vi "RTTrapTest-05-2017.vi"() -> ()   [LabVIEW 2010]
uses:
  <vilib>/rvi/interface/nirviOpenFPGA/nirviOpenFPGA.xnode
  <vilib>/userDefined/High Color/nirio_resource_hc.ctl
  <vilib>/rvi/interface/nirviReadWriteControl/nirviReadWriteControl.xnode
  <vilib>/Utility/error.llb/Error Cluster From Error Code.vi
  <vilib>/rvi/errors/niLvFpgaWhatHappensToTopLevelVI.ctl
  <vilib>/rvi/interface/common/niFpgaNodeNameForErrorReporting.ctl
  <vilib>/rvi/errors/niLvFpgaAdjustHostInterfaceError.vi
  <vilib>/rvi/interface/nirviMethod/nirviMethod.xnode
  NiFpgaLv.dll
  <vilib>/rvi/interface/nirviCloseFPGA/nirviCloseFPGA.xnode
  C:/Users/HAGAR-IV/Desktop/Zeugs/markus/version feb 2012/FPGA Bitfiles/pertrasgcfpga2_FPGATarget_FPGA-TrapTest-05_C2F74D86.lvbitx
  C:/Users/HAGAR-IV/Desktop/Zeugs/Johnny/pertrasgc fpga/FPGA-TrapTest-05-2017.vi
  <vilib>/FPGAPlugInAG/cRIO-9114/niLvFpga_Open_cRIO-9114.vi
  <vilib>/rvi/ClientSDK/nirviWhatTheDeviceIsDoing.ctl
  <vilib>/RVI Host/nirviSupport.llb/nirviErrorClusterFromErrorCode.vi
  <vilib>/FPGAPlugInAG/cRIO-9114/niLvFpga_Close_cRIO-9114.vi
panel:
  in  "Vorlaufzeit":dbl
  in  "Heizung aus":bool
  out "Uhr":dbl
  in  "Heizen&Starten":bool
  in  "Rampenende":dbl
  in  "T2":dbl
  in  "T1":dbl
  out "ThermoTemp":dbl
  out "PTTempTrap":dbl[](graph)
  in  "ThermoKoeff0":dbl=12.98
  in  "ThermoKoeff2":dbl=-136.78
  in  "ThermoKoeff1":dbl=1284.53
  in  "PTStirlingKoeff0":dbl=-248.3
  in  "PTStirlingKoeff2":dbl=2.42
  in  "PTStirlingKoeff1":dbl=108.05
  in  "SollwertTemp":dbl=50.0
  in  "R(T)Koeff0":dbl=7.31
  in  "R(T)Koeff2":dbl=5.2e-05
  in  "R(T)Koeff1":dbl=0.032
  out "TempTrap":dbl[](graph)
  in  "Löschen":bool
  out "SollwertSchpannung":dbl
  out "SollwertWidrschtond":dbl=8.43
  out "TempTrap":dbl
  in  "T(R)Koeff0":dbl=-236.6
  in  "T(R)Koeff2":dbl=-0.6
  in  "T(R)Koeff1":dbl=37.1
  out "WiderstandHeizdraht":dbl
  out "PTStirling":dbl format="%.2f"
  in  "Stirling":bool
  out "Thermo [V]":fxp<+/-,26,5> format="%.23g"
  in  "Messwerte":i32=10
  in  "Heizen":bool
  in  "5Van(us)":u16=5500
  in  "Periode(us)":u32=100000
  out "Messwert":fxp<+/-,27,6> format="%.23g"
  in  "Warten(us)":u16=5000
  in  "zwischenMesswerten(us)":u16=10
  in  "PID gains":T1={"proportional gain (Kc)"=5.0, "integral gain (Kc*Ts/Ti)"=0.0, "derivative gain (Kc*Td/Ts)"=0.0} {"proportional gain (Kc)" format="%.11g"; "integral gain (Kc*Ts/Ti)" format="%.11g"; "derivative gain (Kc*Td/Ts)" format="%.11g"}
  in  "stop":bool
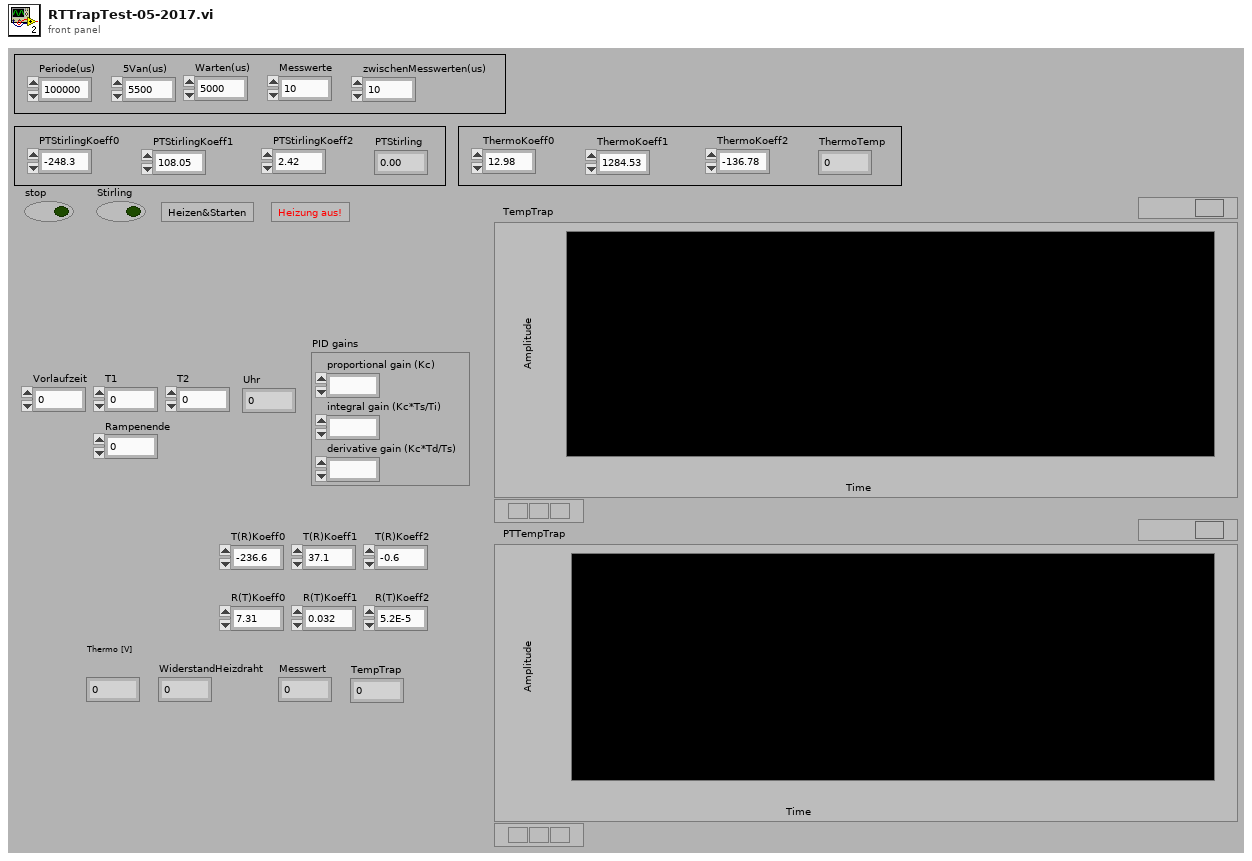
[diagram p1: front panel]
types:
  T1 = cluster{"proportional gain (Kc)":fxp<+/-,16,8>, "integral gain (Kc*Ts/Ti)":fxp<+/-,16,8>, "derivative gain (Kc*Td/Ts)":fxp<+/-,16,8>}
  T2 = typedef "niFpgaNodeNameForErrorReporting.ctl" = enum16{"Open FPGA VI Reference", "Read/Write Control", "Invoke Method: Abort", "Invoke Method: Acknowledge IRQ", "Invoke Method: Download", "Invoke Method: FIFO.Configure", "Invoke Method: FIFO.Read", "Invoke Method: FIFO.Start", "Invoke Method: FIFO.Stop", "Invoke Method: FIFO.Write", "Invoke Method: Reset", "Invoke Method: Run", "Invoke Method: Wait on IRQ", "Close FPGA VI Reference"}
  T3 = typedef "niLvFpgaWhatHappensToTopLevelVI.ctl" = enum16{"top level VI scripted behind XNode", "top level VI inlined behind XNode"}
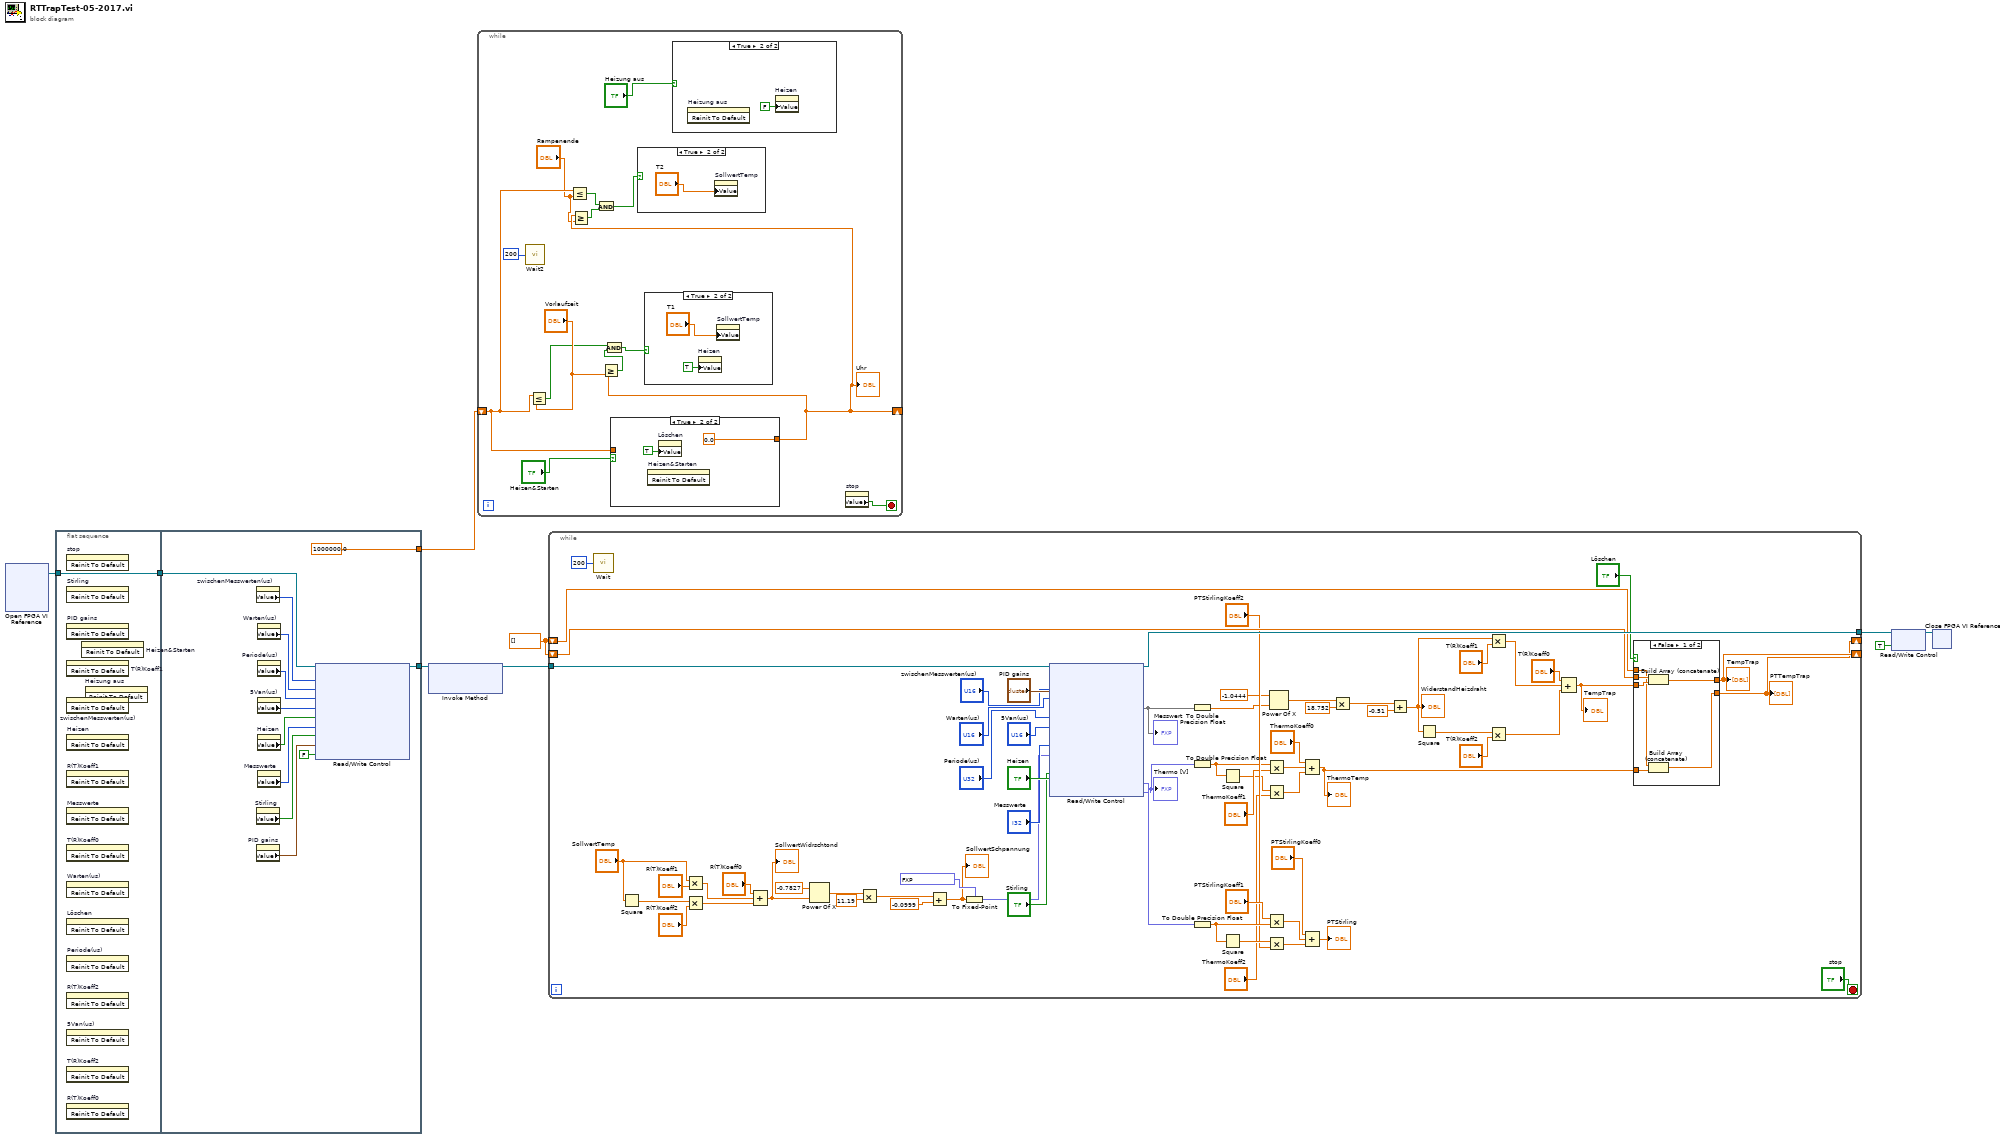
[diagram p0: block diagram]
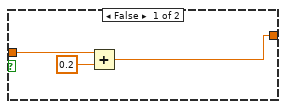
[diagram p5: hidden frame]
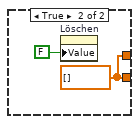
[diagram p6: hidden frame]
diagram:
  w2 = dbl[] []
  n1 = xnode "Open FPGA VI Reference"() -> ("FPGA VI Reference Out"=w9:refnum<k20>)  [unwired: 2 in, 1 out]
  n2 = flat-sequence {
    tunnel: w9 -> [w10]
    tunnel: [w10] -> w3
    tunnel: [w21] -> w8
    tunnel: w3 -> [w22]
    tunnel: [1000000.0] -> w1
    frame #0 {
      n3 = invoke on="stop" class="Bool (strict)" method="Reinit To Default"() -> ()  [unwired: 3 in, 3 out]
      n4 = invoke on="Stirling" class="Bool (strict)" method="Reinit To Default"() -> ()  [unwired: 3 in, 3 out]
      n5 = invoke on="PID gains" class="Clust (strict)" method="Reinit To Default"() -> ()  [unwired: 3 in, 3 out]
      n6 = invoke on="T(R)Koeff1" class="DigNum (strict)" method="Reinit To Default"() -> ()  [unwired: 3 in, 3 out]
      n7 = invoke on="zwischenMesswerten(us)" class="DigNum (strict)" method="Reinit To Default"() -> ()  [unwired: 3 in, 3 out]
      n8 = invoke on="Heizen" class="Bool (strict)" method="Reinit To Default"() -> ()  [unwired: 3 in, 3 out]
      n9 = invoke on="R(T)Koeff1" class="DigNum (strict)" method="Reinit To Default"() -> ()  [unwired: 3 in, 3 out]
      n10 = invoke on="Messwerte" class="DigNum (strict)" method="Reinit To Default"() -> ()  [unwired: 3 in, 3 out]
      n11 = invoke on="T(R)Koeff0" class="DigNum (strict)" method="Reinit To Default"() -> ()  [unwired: 3 in, 3 out]
      n12 = invoke on="Warten(us)" class="DigNum (strict)" method="Reinit To Default"() -> ()  [unwired: 3 in, 3 out]
      n13 = invoke on="Löschen" class="Bool (strict)" method="Reinit To Default"() -> ()  [unwired: 3 in, 3 out]
      n14 = invoke on="Periode(us)" class="DigNum (strict)" method="Reinit To Default"() -> ()  [unwired: 3 in, 3 out]
      n15 = invoke on="R(T)Koeff2" class="DigNum (strict)" method="Reinit To Default"() -> ()  [unwired: 3 in, 3 out]
      n16 = invoke on="5Van(us)" class="DigNum (strict)" method="Reinit To Default"() -> ()  [unwired: 3 in, 3 out]
      n17 = invoke on="T(R)Koeff2" class="DigNum (strict)" method="Reinit To Default"() -> ()  [unwired: 3 in, 3 out]
      n18 = invoke on="R(T)Koeff0" class="DigNum (strict)" method="Reinit To Default"() -> ()  [unwired: 3 in, 3 out]
      n19 = invoke on="Heizen&Starten" class="Bool" method="Reinit To Default"() -> ()  [unwired: 3 in, 3 out]
      n20 = invoke on="Heizung aus" class="Bool" method="Reinit To Default"() -> ()  [unwired: 3 in, 3 out]
    }
    frame #1 {
      n21 = property on="zwischenMesswerten(us)" class="DigNum (strict)"() -> ("Value"=w20:u16)  [unwired: 2 in, 2 out]
      n22 = property on="Stirling" class="Bool (strict)"() -> ("Value"=w14:bool)  [unwired: 2 in, 2 out]
      n23 = property on="PID gains" class="Clust (strict)"() -> ("Value"=w13:T1)  [unwired: 2 in, 2 out]
      n24 = property on="Warten(us)" class="DigNum (strict)"() -> ("Value"=w19:u16)  [unwired: 2 in, 2 out]
      n25 = property on="Periode(us)" class="DigNum (strict)"() -> ("Value"=w18:u32)  [unwired: 2 in, 2 out]
      n26 = property on="5Van(us)" class="DigNum (strict)"() -> ("Value"=w17:u16)  [unwired: 2 in, 2 out]
      n27 = property on="Heizen" class="Bool (strict)"() -> ("Value"=w16:bool)  [unwired: 2 in, 2 out]
      n28 = property on="Messwerte" class="DigNum (strict)"() -> ("Value"=w15:i32)  [unwired: 2 in, 2 out]
      n29 = xnode "Read/Write Control"("FPGA VI Reference In"=w22, "zwischenMesswerten(us)"=w20, "Warten(us)"=w19, "Periode(us)"=w18, "5Van(us)"=w17, "HeizenTrap1"=w16, "Messwerte"=w15, "Stirling"=w14, "PIDTrap1"=w13, "stop"=FALSE) -> ("FPGA VI Reference Out"=w21:refnum<k20>)  [unwired: 1 in, 1 out]
    }
  }
  n30 = xnode "Invoke Method"("FPGA VI Reference In"=w8) -> ("FPGA VI Reference Out"=w7:refnum<k20>)  [unwired: 2 in, 1 out]
  n31 = while {
    shift-right: [w234] -> _
    shift-left: w1 -> [w235]
    stop <- w241 stop-if-true
    n32 = call "Wait2"("Count(mSec)"=u32 200) -> ()  [unwired: 1 out]
    n33 = Less Or Equal?(x=w235, y="Vorlaufzeit") -> (x <= y?=w237:bool)
    n34 = Less Or Equal?(x=w235, y="Rampenende") -> (x <= y?=w232:bool)
    n35 = case shown="True" "Heizen&Starten" {
      tunnel: w235 -> [w249 _]
      tunnel: [w247 0.0 ("t")] -> w234
      frame False {
        n36 = Add(x=w249, y=0.2) -> (x+y=w247:dbl)
      }
      frame True {
        n37 = invoke on="Heizen&Starten" class="Bool" method="Reinit To Default"() -> ()  [unwired: 3 in, 3 out]
        n38 = property on="Löschen" class="Bool (strict)"("Value"=TRUE ("Löschen")) -> ()  [unwired: 2 in, 2 out]
      }
    }
    "Uhr" <- w234
    n39 = Greater Or Equal?(x=w234, y="Rampenende") -> (x >= y?=w231:bool)
    n40 = And(x=w232, y=w231) -> (x .and. y?=w230:bool)
    n41 = Greater Or Equal?(x=w234, y="Vorlaufzeit") -> (x >= y?=w238:bool)
    n42 = And(x=w237, y=w238) -> (x .and. y?=w236:bool)
    n43 = case shown="True" w230 {
      frame False {
      }
      frame True {
        n44 = property on="SollwertTemp" class="DigNum (strict)"("Value"="T2") -> ()  [unwired: 2 in, 2 out]
      }
    }
    n45 = case shown="True" w236 {
      frame False {
      }
      frame True {
        n46 = property on="Heizen" class="Bool (strict)"("Value"=TRUE ("Heizen")) -> ()  [unwired: 2 in, 2 out]
        n47 = property on="SollwertTemp" class="DigNum (strict)"("Value"="T1") -> ()  [unwired: 2 in, 2 out]
      }
    }
    n48 = case shown="True" "Heizung aus" {
      frame False {
      }
      frame True {
        n49 = invoke on="Heizung aus" class="Bool" method="Reinit To Default"() -> ()  [unwired: 3 in, 3 out]
        n50 = property on="Heizen" class="Bool (strict)"("Value"=FALSE ("Heizen")) -> ()  [unwired: 2 in, 2 out]
      }
    }
    n51 = property on="stop" class="Bool (strict)"() -> ("Value"=w241:bool)  [unwired: 2 in, 2 out]
  }
  n52 = while {
    tunnel: w7 -> [w317]
    tunnel: [w315] -> w6
    shift-right: [w293] -> _
    shift-left: w2 -> [w295]
    shift-right: [w267] -> _
    shift-left: w2 -> [w276]
    stop <- "stop" stop-if-true
    n53 = call "Wait"("Count(mSec)"=u32 200) -> ()  [unwired: 1 out]
    n54 = Square(x="SollwertTemp") -> (x^2=w292:dbl)
    n55 = Multiply(x="SollwertTemp", y="R(T)Koeff1") -> (x*y=w287:dbl)
    n56 = Multiply(x=w292, y="R(T)Koeff2") -> (x*y=w286:dbl)
    n57 = Compound Arithmetic op=ADD("R(T)Koeff0", w287, w286) -> (w261:dbl)
    "SollwertWidrschtond" <- w261
    n58 = Power Of X(1:w261, 2:-0.7827 ("y")) -> (0:w257:dbl)
    n59 = Multiply(x=w257, y=11.19) -> (x*y=w255:dbl)
    n60 = Add(x=w255, y=-0.0999) -> (x+y=w253:dbl)
    "SollwertSchpannung" <- w253
    n61 = To Fixed-Point(fixed-point type=fxp<+/-,16,6> 0.0 ("setpoint"), number=w253) -> (fixed-point=w298:fxp<+/-,16,6>)
    n62 = xnode "Read/Write Control"("FPGA VI Reference In"=w317, "PID gains"="PID gains", "zwischenMesswerten(us)"="zwischenMesswerten(us)", "Warten(us)"="Warten(us)", "Periode(us)"="Periode(us)", "5Van(us)"="5Van(us)", "Heizen"="Heizen", "Messwerte"="Messwerte", "setpoint"=w298, "Stirling"="Stirling") -> ("FPGA VI Reference Out"=w315:refnum<k20>, "Messwert"=w300, "PTStirling"=w278:fxp<+/-,26,5>, "Thermoelement"=w252:fxp<+/-,26,5>)  [unwired: 1 in, 2 out]
    "Messwert" <- w300
    "Thermo [V]" <- w252
    n63 = To Double Precision Float(number=w300) -> (double precision float=w260:dbl)
    n64 = To Double Precision Float(number=w252) -> (double precision float=w272:dbl)
    n65 = To Double Precision Float(number=w278) -> (double precision float=w284:dbl)
    n66 = Square(x=w272) -> (x^2=w271:dbl)
    n67 = Square(x=w284) -> (x^2=w283:dbl)
    n68 = Multiply(x=w272, y="ThermoKoeff1") -> (x*y=w273:dbl)
    n69 = Multiply(x=w271, y="ThermoKoeff2") -> (x*y=w269:dbl)
    n70 = Multiply(x="PTStirlingKoeff1", y=w284) -> (x*y=w280:dbl)
    n71 = Multiply(x=w283, y="PTStirlingKoeff2") -> (x*y=w279:dbl)
    n72 = Power Of X(1:w260, 2:-1.0444 ("x")) -> (0:w266:dbl)
    n73 = Compound Arithmetic op=ADD("ThermoKoeff0", w273, w269) -> (w268:dbl)
    "ThermoTemp" <- w268
    n74 = Compound Arithmetic op=ADD("PTStirlingKoeff0", w280, w279) -> (→"PTStirling":dbl)
    n75 = Multiply(x=w266, y=18.752) -> (x*y=w264:dbl)
    n76 = Add(x=w264, y=-0.51) -> (x+y=w262:dbl)
    "WiderstandHeizdraht" <- w262
    n77 = Square(x=w262) -> (x^2=w305:dbl)
    n78 = Multiply(x=w262, y="T(R)Koeff1") -> (x*y=w302:dbl)
    n79 = Multiply(x=w305, y="T(R)Koeff2") -> (x*y=w303:dbl)
    n80 = Compound Arithmetic op=ADD("T(R)Koeff0", w302, w303) -> (w296:dbl)
    "TempTrap" <- w296
    n81 = case shown="False" "Löschen" {
      tunnel: w296 -> [w323 _]
      tunnel: [w322 w324] -> w293
      tunnel: w295 -> [w321 _]
      tunnel: [w320 w324] -> w267
      tunnel: w276 -> [w319 _]
      tunnel: w268 -> [w318 _]
      frame False {
        n82 = Build Array (concatenate)(w321, w323) -> (w322:dbl[])
        n83 = Build Array (concatenate)(w319, w318) -> (w320:dbl[])
      }
      frame True {
        w324 = dbl[] []
        n84 = property on="Löschen" class="Bool (strict)"("Value"=FALSE ("Löschen")) -> ()  [unwired: 2 in, 2 out]
      }
    }
    "TempTrap" <- w293
    "PTTempTrap" <- w267
  }
  n85 = xnode "Read/Write Control"("FPGA VI Reference In"=w6, "stop"=TRUE) -> ("FPGA VI Reference Out"=w4:refnum<k20>)  [unwired: 1 in, 1 out]
  n86 = xnode "Close FPGA VI Reference"("FPGA VI Reference In"=w4) -> ()  [unwired: 1 in, 1 out]
